vi "supervision Feux.vi"() -> ()   [LabVIEW 2013]
uses:
  <vilib>/Instr/_visa.llb/VISA Configure Serial Port (Instr).vi
panel:
  in  "?":T1(tab)
  in  "?":bool
  in  "?":enum32{"Voie 1", ""}(radio)
  in  "?":enum32{"Voie 2", ""}(radio)
  in  "?":enum32{"Voie 3", ""}(radio)
  in  "?":enum32{"Voie 4", ""}(radio)
  in  "Temporisation Vert (en seconde)":dbl=3.0
  in  "Temporisation Jaune  (en seconde)":dbl=2.0
  in  "Temporisation Rouge (en seconde)":dbl=1.0
  in  "?":bool
  in  "Temporisation Vert 4":dbl=3.0
  in  "Temporisation Jaune":dbl=2.0
  in  "Temporisation Rouge":dbl=1.0
  in  "Temporisation Vert 3":dbl=3.0
  in  "Temporisation Jaune  2":dbl=2.0
  in  "Temporisation Rouge":dbl=1.0
  in  "Temporisation Vert 2":dbl=3.0
  in  "Temporisation Jaune  2":dbl=2.0
  in  "Temporisation Rouge":dbl=1.0
  in  "Temporisation Vert":dbl=3.0
  in  "Temporisation Jaune":dbl=2.0
  in  "Temporisation Rouge":dbl=1.0
  in  "?":bool
  out "valeur sélectionnée":string
  in  "?":bool
  out "sortie d'erreur":errorcluster
  in  "entrée d'erreur":errorcluster caption="entrée d'erreur (pas d'erreur)"
  in  "VISA resource name":refnum<visa-resource-name> caption="Arduino connectée sur sortie USB"
  out "?":bool
  out "?":bool
  out "?":bool
  out "?":bool
  out "?":bool
  out "?":bool
  out "?":bool
  out "?":bool
  out "?":bool
  out "?":bool
  out "?":bool
  out "?":bool
  # "ECRAN DE SUPERVISION DU CARREFOUR 1"
  # "VOIE 1"
  # "VOIE 4"
  # "VOIE 2"
  # "VOIE 3"
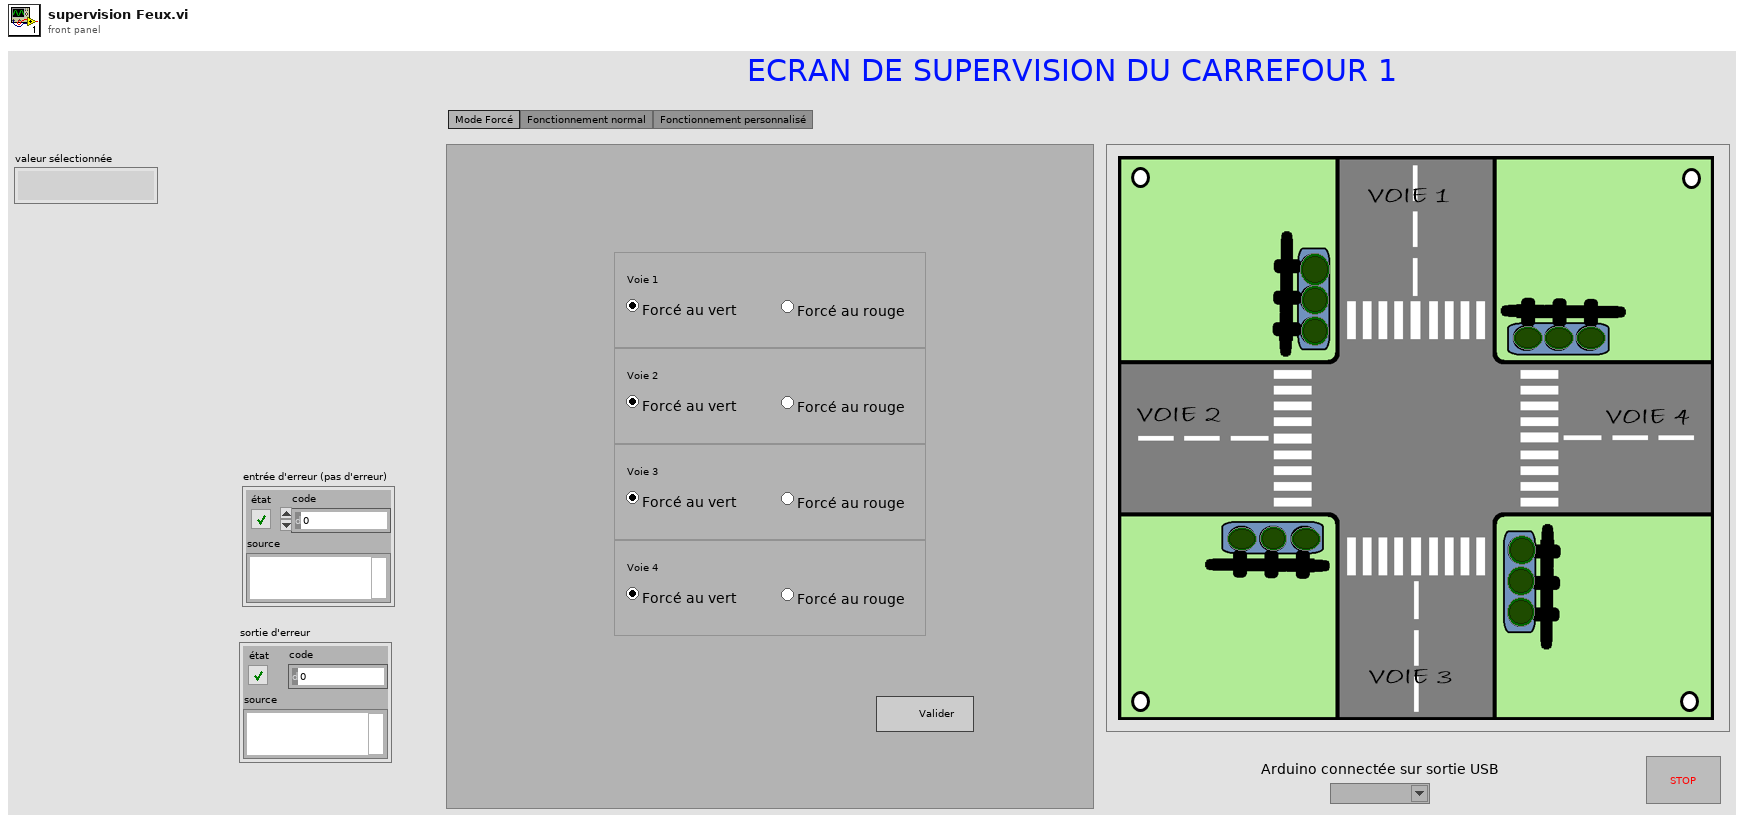
[diagram p1: front panel]
types:
  T1 = enum32{"Mode Forcé", "Fonctionnement normal", "Fonctionnement personnalisé"}
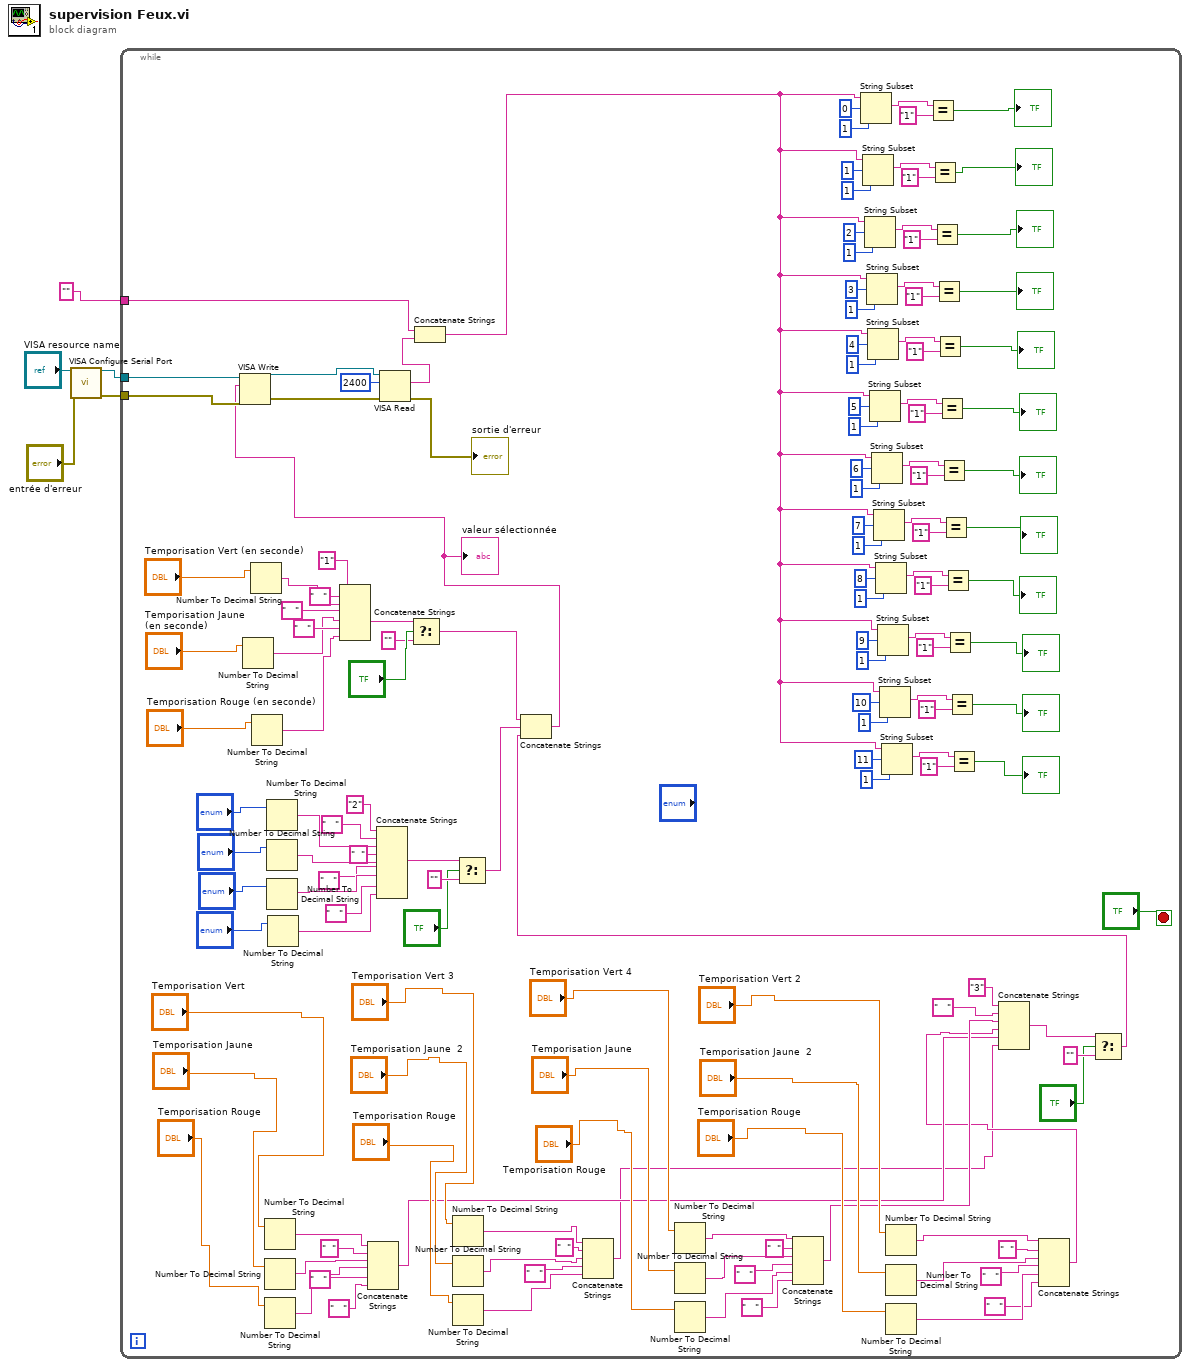
[diagram p0: block diagram]
diagram:
  n1 = call-poly "VISA Configure Serial Port"("VISA resource name"="VISA resource name", "error in (no error)"="entrée d'erreur") -> ("VISA resource name out"=w5:refnum<visa-resource-name>, "error out"=w2:errorcluster)  [unwired: 12 in]
  n2 = while {
    tunnel: w5 -> [w150]
    tunnel: "" -> [w149]
    tunnel: w2 -> [w90]
    stop <- "?" stop-if-true
    n3 = Number To Decimal String(number="Temporisation Jaune  (en seconde)") -> (decimal integer string=w76:string)  [unwired: 1 in]
    n4 = Number To Decimal String(number="Temporisation Vert (en seconde)") -> (decimal integer string=w77:string)  [unwired: 1 in]
    n5 = Number To Decimal String(number="Temporisation Rouge (en seconde)") -> (decimal integer string=w75:string)  [unwired: 1 in]
    n6 = Number To Decimal String(number="Temporisation Vert") -> (decimal integer string=w44:string)  [unwired: 1 in]
    n7 = Number To Decimal String(number="Temporisation Jaune") -> (decimal integer string=w43:string)  [unwired: 1 in]
    n8 = Number To Decimal String(number="Temporisation Rouge") -> (decimal integer string=w42:string)  [unwired: 1 in]
    n9 = Number To Decimal String(number="?") -> (decimal integer string=w74:string)  [unwired: 1 in]
    n10 = Number To Decimal String(number="?") -> (decimal integer string=w72:string)  [unwired: 1 in]
    n11 = Number To Decimal String(number="?") -> (decimal integer string=w71:string)  [unwired: 1 in]
    n12 = Number To Decimal String(number="?") -> (decimal integer string=w70:string)  [unwired: 1 in]
    n13 = Concatenate Strings("1" ("chaîne"), "   " ("chaîne"), w77, "   " ("chaîne"), w76, "   " ("chaîne"), w75) -> (w87:string)
    n14 = Concatenate Strings(w44, "  " ("chaîne"), w43, "   " ("chaîne"), w42, "   " ("chaîne")) -> (w9:string)
    n15 = Concatenate Strings("2" ("chaîne"), "   " ("chaîne"), w74, "  " ("chaîne"), w72, "   " ("chaîne"), w71, "   " ("chaîne"), w70) -> (w63:string)
    n16 = Select(t=w87, s="?", f="" ("cas faux")) -> (s? t:f=w60:string)
    n17 = Number To Decimal String(number="Temporisation Vert 3") -> (decimal integer string=w40:string)  [unwired: 1 in]
    n18 = Number To Decimal String(number="Temporisation Jaune  2") -> (decimal integer string=w39:string)  [unwired: 1 in]
    n19 = Number To Decimal String(number="Temporisation Rouge") -> (decimal integer string=w38:string)  [unwired: 1 in]
    n20 = Select(t=w63, s="?", f="" ("cas faux")) -> (s? t:f=w59:string)
    n21 = Concatenate Strings(w40, "  " ("chaîne"), w39, "   " ("chaîne"), w38) -> (w7:string)
    n22 = Number To Decimal String(number="Temporisation Vert 4") -> (decimal integer string=w37:string)  [unwired: 1 in]
    n23 = Number To Decimal String(number="Temporisation Jaune") -> (decimal integer string=w36:string)  [unwired: 1 in]
    n24 = Number To Decimal String(number="Temporisation Rouge") -> (decimal integer string=w35:string)  [unwired: 1 in]
    n25 = Concatenate Strings(w37, "  " ("chaîne"), w36, "   " ("chaîne"), w35, "   " ("chaîne")) -> (w10:string)
    n26 = Number To Decimal String(number="Temporisation Vert 2") -> (decimal integer string=w34:string)  [unwired: 1 in]
    n27 = Number To Decimal String(number="Temporisation Jaune  2") -> (decimal integer string=w33:string)  [unwired: 1 in]
    n28 = Number To Decimal String(number="Temporisation Rouge") -> (decimal integer string=w32:string)  [unwired: 1 in]
    n29 = Concatenate Strings(w34, "  " ("chaîne"), w33, "   " ("chaîne"), w32, "   " ("chaîne")) -> (w8:string)
    n30 = Concatenate Strings("3" ("chaîne"), "   " ("chaîne"), w10, w8, w9, w7) -> (w56:string)
    n31 = Select(t=w56, s="?", f="" ("cas faux")) -> (s? t:f=w54:string)
    n32 = Concatenate Strings(w60, w59, w54) -> (w55:string)
    "valeur sélectionnée" <- w55
    n33 = VISA Write(VISA resource name=w150, write buffer=w55, error in (no error)=w90) -> (VISA resource name out=w151:refnum<visa-resource-name>, error out=w92:errorcluster)  [unwired: 1 out]
    n34 = VISA Read(VISA resource name=w151, byte count=u32 2400 ("nombre d'octets"), error in (no error)=w92) -> (read buffer=w148:string, error out=→"sortie d'erreur":errorcluster)  [unwired: 2 out]
    n35 = Concatenate Strings(w149, w148) -> (w97:string)
    n36 = String Subset(string=w97, offset (0)=0, length (rest)=1 ("longueur (reste)")) -> (substring=w144:string)
    n37 = String Subset(string=w97, offset (0)=1, length (rest)=1 ("longueur (reste)")) -> (substring=w140:string)
    n38 = String Subset(string=w97, offset (0)=2, length (rest)=1 ("longueur (reste)")) -> (substring=w137:string)
    n39 = String Subset(string=w97, offset (0)=3, length (rest)=1 ("longueur (reste)")) -> (substring=w133:string)
    n40 = String Subset(string=w97, offset (0)=4, length (rest)=1 ("longueur (reste)")) -> (substring=w129:string)
    n41 = String Subset(string=w97, offset (0)=5, length (rest)=1 ("longueur (reste)")) -> (substring=w125:string)
    n42 = String Subset(string=w97, offset (0)=6, length (rest)=1 ("longueur (reste)")) -> (substring=w121:string)
    n43 = String Subset(string=w97, offset (0)=7, length (rest)=1 ("longueur (reste)")) -> (substring=w117:string)
    n44 = String Subset(string=w97, offset (0)=8, length (rest)=1 ("longueur (reste)")) -> (substring=w113:string)
    n45 = String Subset(string=w97, offset (0)=9, length (rest)=1 ("longueur (reste)")) -> (substring=w109:string)
    n46 = String Subset(string=w97, offset (0)=10, length (rest)=1 ("longueur (reste)")) -> (substring=w105:string)
    n47 = String Subset(string=w97, offset (0)=11, length (rest)=1 ("longueur (reste)")) -> (substring=w101:string)
    n48 = Equal?(x=w144, y="1") -> (x = y?=→"?":bool)
    n49 = Equal?(x=w140, y="1") -> (x = y?=→"?":bool)
    n50 = Equal?(x=w137, y="1") -> (x = y?=→"?":bool)
    n51 = Equal?(x=w133, y="1") -> (x = y?=→"?":bool)
    n52 = Equal?(x=w129, y="1") -> (x = y?=→"?":bool)
    n53 = Equal?(x=w125, y="1") -> (x = y?=→"?":bool)
    n54 = Equal?(x=w121, y="1") -> (x = y?=→"?":bool)
    n55 = Equal?(x=w117, y="1") -> (x = y?=→"?":bool)
    n56 = Equal?(x=w113, y="1") -> (x = y?=→"?":bool)
    n57 = Equal?(x=w109, y="1") -> (x = y?=→"?":bool)
    n58 = Equal?(x=w105, y="1") -> (x = y?=→"?":bool)
    n59 = Equal?(x=w101, y="1") -> (x = y?=→"?":bool)
  }
